vi "RESP3 Format Message.vi"(8 "error in (no error)":errorcluster, 11 "RESP3 Value":variant) -> (0 "error out":errorcluster, 3 "messages":string[](array[string]))   [LabVIEW 2019, in "RESP3.lvlib"]
doc: "<b>Description</b> This VI formats a RESP3 Value into an array of strings that represent the input value. The output of this VI is suitable to send to a peer over a TCP connection.\n\n<b>Inputs</b>\n<b>RESP3 Value</b>: Any valid RESP3 value.\n\n<b>Outputs</b>\n<b>messages</b>: An array of \\r\\n terminated messages that represent the input value.\n\nBSD 3-Clause License\n\nCopyright (c) 2021, TauTerra, LLC\nAll rights reserved.\n\nRedistribution and use in source and binary forms, with or without\nmodification, are permitted provided that the following conditions are met:\n\n1. Redistributions of source code must retain the above copyright notice, this\n list of conditions and the following disclaimer.\n\n2. Redistributions in binary form must reproduce the above copyright notice,\n this list of conditions and the following disclaimer in the documentation\n and/or other materials provided with the distribution.\n\n3. Neither the name of the copyright holder nor the names of its\n contributors may be used to endorse or promote products derived from\n this software without specific prior written permission.\n\nTHIS SOFTWARE IS PROVIDED BY THE COPYRIGHT HOLDERS AND CONTRIBUTORS \"AS IS\"\nAND ANY EXPRESS OR IMPLIED WARRANTIES, INCLUDING, BUT NOT LIMITED TO, THE\nIMPLIED WARRANTIES OF MERCHANTABILITY AND FITNESS FOR A PARTICULAR PURPOSE ARE\nDISCLAIMED. IN NO EVENT SHALL THE COPYRIGHT HOLDER OR CONTRIBUTORS BE LIABLE\nFOR ANY DIRECT, INDIRECT, INCIDENTAL, SPECIAL, EXEMPLARY, OR CONSEQUENTIAL\nDAMAGES (INCLUDING, BUT NOT LIMITED TO, PROCUREMENT OF SUBSTITUTE GOODS OR\nSERVICES; LOSS OF USE, DATA, OR PROFITS; OR BUSINESS INTERRUPTION) HOWEVER\nCAUSED AND ON ANY THEORY OF LIABILITY, WHETHER IN CONTRACT, STRICT LIABILITY,\nOR TORT (INCLUDING NEGLIGENCE OR OTHERWISE) ARISING IN ANY WAY OUT OF THE USE\nOF THIS SOFTWARE, EVEN IF ADVISED OF THE POSSIBILITY OF SUCH DAMAGE."
uses:
  RESP3.lvlib
  types/RESP3 data type attribute.vi
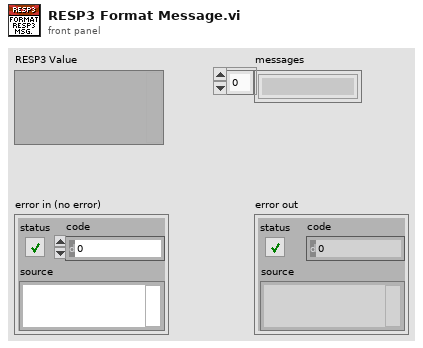
[diagram p1: front panel]
types:
  T1 = typedef "RESP3.lvlib/RESP3 Type.ctl" = enum8{"<0x00>", "<0x01>", "<0x02>", "<0x03>", "<0x04>", "<0x05>", "<0x06>", "<0x07>", "<0x08>", "<0x09>", "<0x0A>", "<0x0B>", "<0x0C>", "<0x0D>", "<0x0E>", "<0x0F>", "<0x10>", "<0x11>", "<0x12>", "<0x13>", "<0x14>", "<0x15>", "<0x16>", "<0x17>", "<0x18>", "<0x19>", "<0x1A>", "<0x1B>", "<0x1C>", "<0x1D>", "<0x1E>", "<0x1F>", "\" \"", "BLOB ERROR", "\"\"\"", "BOOLEAN", "BLOB", "MAP", "\"&\"", "\"'\"", "BIG NUMBER", "\")\"", "ARRAY", "STRING", "DOUBLE", "ERROR", "END", "\"/\"", "\"0\"", "\"1\"", "\"2\"", "\"3\"", "\"4\"", "\"5\"", "\"6\"", "\"7\"", "\"8\"", "\"9\"", "INTEGER", "STREAM", "\"<\"", "VERBATIM STRING", "PUSH", "\"?\"", "\"@\"", "\"A\"", "\"B\"", "\"C\"", "\"D\"", "\"E\"", "\"F\"", "\"G\"", "\"H\"", "\"I\"", "\"J\"", "\"K\"", "\"L\"", "\"M\"", "\"N\"", "\"O\"", "\"P\"", "\"Q\"", "\"R\"", "\"S\"", "\"T\"", "\"U\"", "\"V\"", "\"W\"", "\"X\"", "\"Y\"", "\"Z\"", "\"[\"", "\"\\\"", "\"]\"", "\"^\"", "NULL", "\"`\"", "\"a\"", "\"b\"", "\"c\"", "\"d\"", "\"e\"", "\"f\"", "\"g\"", "\"h\"", "\"i\"", "\"j\"", "\"k\"", "\"l\"", "\"m\"", "\"n\"", "\"o\"", "\"p\"", "\"q\"", "\"r\"", "\"s\"", "\"t\"", "\"u\"", "\"v\"", "\"w\"", "\"x\"", "\"y\"", "\"z\"", "\"{\"", "ATTRIBUTES", "\"}\"", "SET", "<0x7F>", "<0x80>", "<0x81>", "<0x82>", "<0x83>", "<0x84>", "<0x85>", "<0x86>", "<0x87>", "<0x88>", "<0x89>", "<0x8A>", "<0x8B>", "<0x8C>", "<0x8D>", "<0x8E>", "<0x8F>", "<0x90>", "<0x91>", "<0x92>", "<0x93>", "<0x94>", "<0x95>", "<0x96>", "<0x97>", "<0x98>", "<0x99>", "<0x9A>", "<0x9B>", "<0x9C>", "<0x9D>", "<0x9E>", "<0x9F>", "<0xA0>", "<0xA1>", "<0xA2>", "<0xA3>", "<0xA4>", "<0xA5>", "<0xA6>", "<0xA7>", "<0xA8>", "<0xA9>", "<0xAA>", "<0xAB>", "<0xAC>", "<0xAD>", "<0xAE>", "<0xAF>", "<0xB0>", "<0xB1>", "<0xB2>", "<0xB3>", "<0xB4>", "<0xB5>", "<0xB6>", "<0xB7>", "<0xB8>", "<0xB9>", "<0xBA>", "<0xBB>", "<0xBC>", "<0xBD>", "<0xBE>", "<0xBF>", "<0xC0>", "<0xC1>", "<0xC2>", "<0xC3>", "<0xC4>", "<0xC5>", "<0xC6>", "<0xC7>", "<0xC8>", "<0xC9>", "<0xCA>", "<0xCB>", "<0xCC>", "<0xCD>", "<0xCE>", "<0xCF>", "<0xD0>", "<0xD1>", "<0xD2>", "<0xD3>", "<0xD4>", "<0xD5>", "<0xD6>", "<0xD7>", "<0xD8>", "<0xD9>", "<0xDA>", "<0xDB>", "<0xDC>", "<0xDD>", "<0xDE>", "<0xDF>", "<0xE0>", "<0xE1>", "<0xE2>", "<0xE3>", "<0xE4>", "<0xE5>", "<0xE6>", "<0xE7>", "<0xE8>", "<0xE9>", "<0xEA>", "<0xEB>", "<0xEC>", "<0xED>", "<0xEE>", "<0xEF>", "<0xF0>", "<0xF1>", "<0xF2>", "<0xF3>", "<0xF4>", "<0xF5>", "<0xF6>", "<0xF7>", "<0xF8>", "<0xF9>", "<0xFA>", "<0xFB>", "<0xFC>", "<0xFD>", "<0xFE>"}
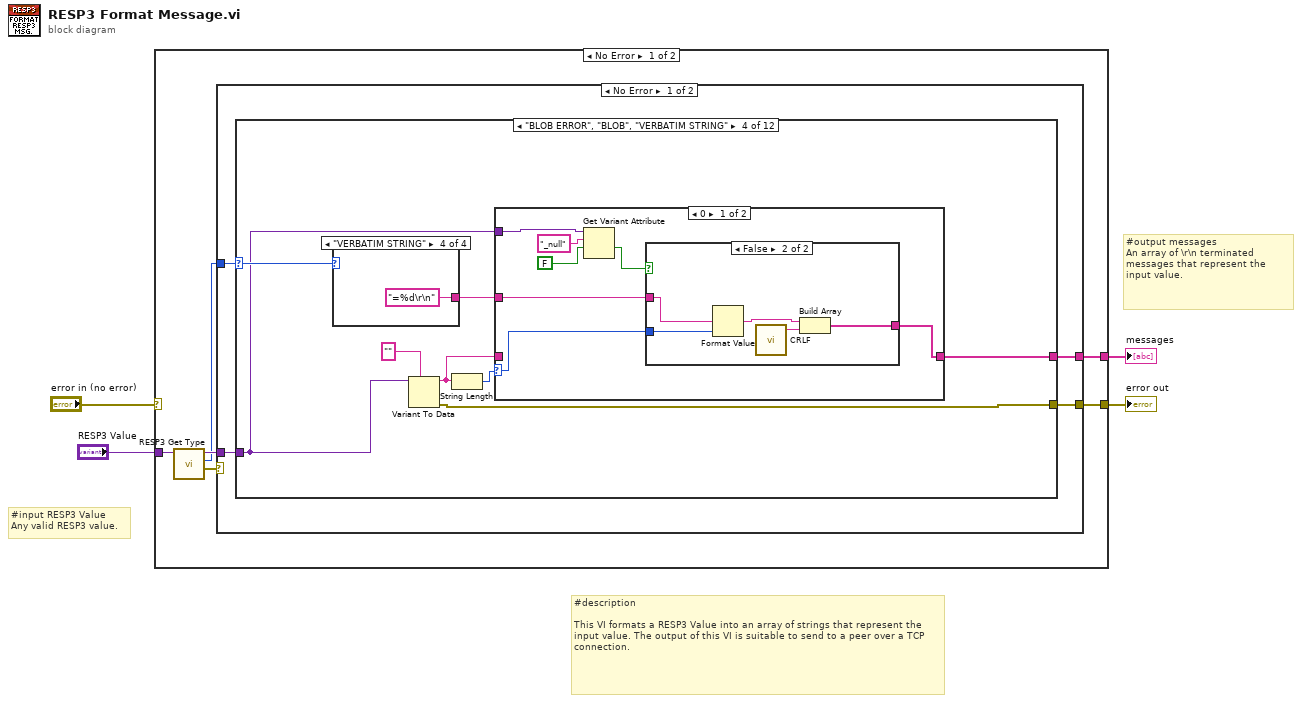
[diagram p0: block diagram]
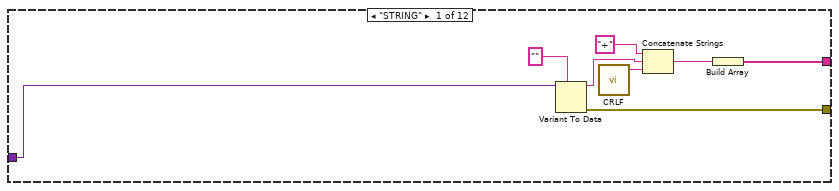
[diagram p2: hidden frame]
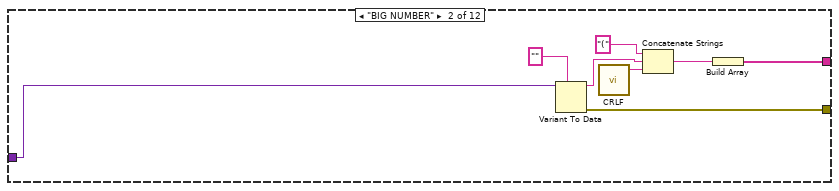
[diagram p3: hidden frame]
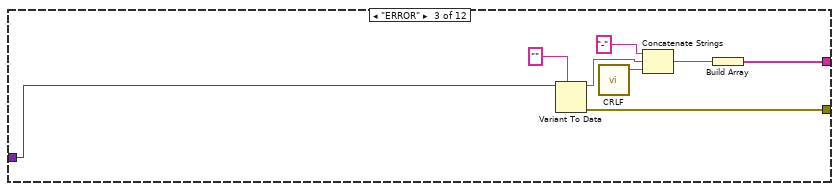
[diagram p4: hidden frame]
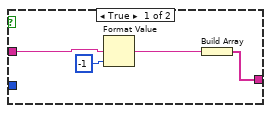
[diagram p5: hidden frame]
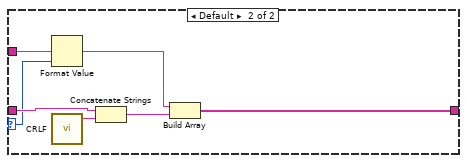
[diagram p6: hidden frame]
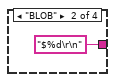
[diagram p8: hidden frame]
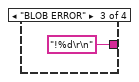
[diagram p9: hidden frame]
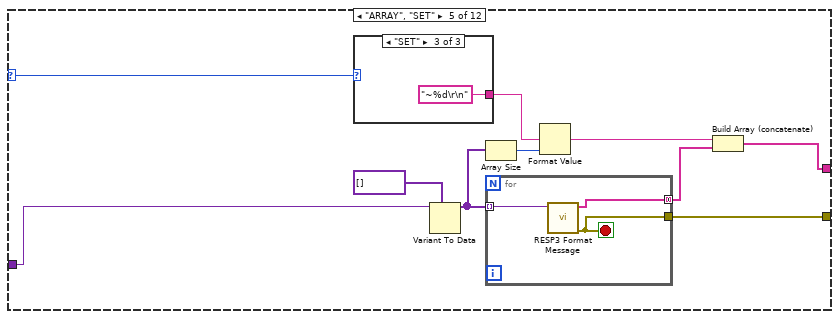
[diagram p10: hidden frame]
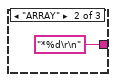
[diagram p12: hidden frame]
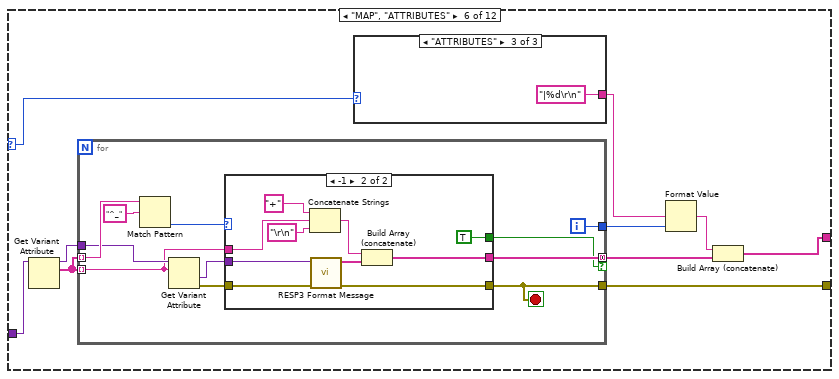
[diagram p13: hidden frame]
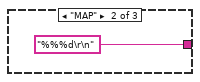
[diagram p15: hidden frame]
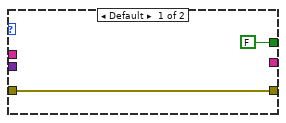
[diagram p16: hidden frame]
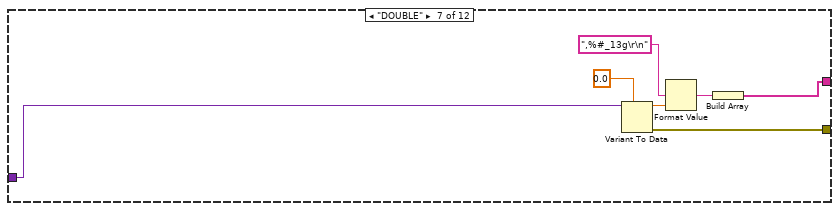
[diagram p17: hidden frame]
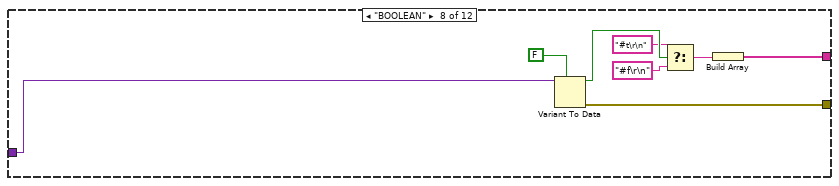
[diagram p18: hidden frame]
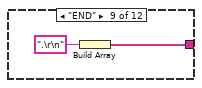
[diagram p19: hidden frame]
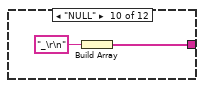
[diagram p20: hidden frame]
diagram:
  # "#description\n\nThis VI formats a RESP3 Value into an array of strings that represent the input value. The output of this VI is suitable to send to a peer over a TCP connection."
  # "#output messages\nAn array of \\r\\n terminated messages that represent the input value."
  # "#input RESP3 Value\nAny valid RESP3 value."
  n1 = case shown="No Error" "error in (no error)" {
    selector: "error in (no error)" -> [_ w152]
    tunnel: "RESP3 Value" -> [w10 _]
    tunnel: [w8 w152] -> w2
    tunnel: [w5 _] -> w1
    frame No Error {
      n2 = call "RESP3 Get Type.vi"("RESP3 Value in"=w10) -> ("error out"=w9:errorcluster, "RESP3 Type"=w6:T1, "RESP3 Value out"=w7:variant)  [unwired: 7 in, 1 out]
      n3 = case shown="No Error" w9 {
        selector: w9 -> [_ w151]
        tunnel: [w12 w151] -> w8
        tunnel: w7 -> [w13 _]
        tunnel: w6 -> [w14 _]
        tunnel: [w11 _] -> w5
        frame No Error {
          n4 = case shown="\"BLOB ERROR\", \"BLOB\", \"VERBATIM STRING\"" w14 {
            selector: w14 -> [_ _ _ w44 w73 w88 _ _ _ _ _ _]
            tunnel: w13 -> [w22 w30 w38 w39 w81 w92 w129 w137 _ _ w148 _]
            tunnel: [w20 w28 w36 w45 w80 w97 w127 w135 _ _ w146 errorcluster {"status"=TRUE, "code"=6015, "source"="invlaid RESP type"} ("error out")] -> w12
            tunnel: [w15 w23 w31 w43 w78 w95 w126 w130 w138 w140 w143 string[] []] -> w11
            frame "STRING" {
              n5 = Variant To Data(type="", Variant=w22) -> (data=w18:string, error out=w20:errorcluster)  [unwired: 1 in]
              n6 = call "CRLF.vi"() -> ("CRLF"=w19:string)  [unwired: 5 in]
              n7 = Concatenate Strings("+" ("string"), w18, w19) -> (w16:string)
              n8 = Build Array(w16) -> (w15:string[])
            }
            frame "BIG NUMBER" {
              n9 = Variant To Data(type="", Variant=w30) -> (data=w26:string, error out=w28:errorcluster)  [unwired: 1 in]
              n10 = call "CRLF.vi"() -> ("CRLF"=w27:string)  [unwired: 5 in]
              n11 = Concatenate Strings("(" ("string"), w26, w27) -> (w24:string)
              n12 = Build Array(w24) -> (w23:string[])
            }
            frame "ERROR" {
              n13 = Variant To Data(type="", Variant=w38) -> (data=w34:string, error out=w36:errorcluster)  [unwired: 1 in]
              n14 = call "CRLF.vi"() -> ("CRLF"=w35:string)  [unwired: 5 in]
              n15 = Concatenate Strings("-" ("string"), w34, w35) -> (w32:string)
              n16 = Build Array(w32) -> (w31:string[])
            }
            frame "BLOB ERROR", "BLOB", "VERBATIM STRING" {
              n17 = case shown="\"VERBATIM STRING\"" w44 {
                tunnel: [_ "$%d\r\n" ("format string") "!%d\r\n" ("format string") "=%d\r\n" ("format string")] -> w40
                frame Default {
                }
                frame "BLOB" {
                }
                frame "BLOB ERROR" {
                }
                frame "VERBATIM STRING" {
                }
              }
              n18 = Variant To Data(type="", Variant=w39) -> (data=w42:string, error out=w45:errorcluster)  [unwired: 1 in]
              n19 = String Length(string=w42) -> (length=w41:i32)
              n20 = case shown="0" w41 {
                selector: w41 -> [w47 w63]
                tunnel: [w52 w67] -> w43
                tunnel: w42 -> [_ w66]
                tunnel: w40 -> [w53 w65]
                tunnel: w39 -> [w51 _]
                frame 0 {
                  n21 = Get Variant Attribute(Variant=w51, name="_null", default value (empty Variant)=FALSE) -> (value=w48:bool)  [unwired: 1 in, 3 out]
                  n22 = case shown="False" w48 {
                    tunnel: w53 -> [w57 w62]
                    tunnel: [w56 w61] -> w52
                    tunnel: w47 -> [_ w59]
                    frame True {
                      n23 = Format Value(format string=w57, value (0)=-1) -> (output string=w55:string)  [unwired: 1 in]
                      n24 = Build Array(w55) -> (w56:string[])
                    }
                    frame False {
                      n25 = Format Value(format string=w62, value (0)=w59) -> (output string=w60:string)  [unwired: 1 in]
                      n26 = call "CRLF.vi"() -> ("CRLF"=w58:string)  [unwired: 5 in]
                      n27 = Build Array(w60, w58) -> (w61:string[])
                    }
                  }
                }
                frame Default {
                  n28 = Format Value(format string=w65, value (0)=w63) -> (output string=w64:string)  [unwired: 1 in]
                  n29 = call "CRLF.vi"() -> ("CRLF"=w69:string)  [unwired: 5 in]
                  n30 = Concatenate Strings(w66, w69) -> (w68:string)
                  n31 = Build Array(w64, w68) -> (w67:string[])
                }
              }
            }
            frame "ARRAY", "SET" {
              n32 = case shown="\"SET\"" w73 {
                tunnel: [_ "*%d\r\n" ("format string") "~%d\r\n" ("format string")] -> w77
                frame Default {
                }
                frame "ARRAY" {
                }
                frame "SET" {
                }
              }
              n33 = Variant To Data(type=variant[] [], Variant=w81) -> (data=w76:variant[])  [unwired: 1 in, 1 out]
              n34 = Array Size(array=w76) -> (size(s)=w75:i32)
              n35 = for {
                tunnel: w76 -> [w87] mode=indexing
                tunnel: [w86] -> w79 mode=concatenating
                tunnel: [w85] -> w80
                stop <- w85 stop-if-true
                n36 = call "RESP3 Format Message.vi"("RESP3 Value"=w87) -> ("error out"=w85:errorcluster, "messages"=w86:string[])  [unwired: 9 in]
              }
              n37 = Format Value(format string=w77, value (0)=w75) -> (output string=w74:string)  [unwired: 1 in]
              n38 = Build Array (concatenate)(w74, w79) -> (w78:string[])
            }
            frame "MAP", "ATTRIBUTES" {
              n39 = Get Variant Attribute(Variant=w92) -> (duplicate Variant=w90:variant, names=w89:string[])  [unwired: 3 in, 2 out]
              n40 = for {
                tunnel: [w110] -> w96 mode=concatenating if=w105
                tunnel: [w109] -> w97
                tunnel: w89 -> [w108] mode=indexing
                tunnel: [w104] -> w91
                tunnel: w90 -> [w103]
                tunnel: w89 -> [w100] mode=indexing
                i -> [w104]
                stop <- w109 stop-if-true
                n41 = Match Pattern(string=w108, regular expression="^_") -> (offset past match=w106:i32)  [unwired: 1 in, 3 out]
                n42 = Get Variant Attribute(Variant=w103, name=w100) -> (value=w102:variant, error out=w101:errorcluster)  [unwired: 2 in, 2 out]
                n43 = case shown="-1" w106 {
                  tunnel: [_ w117] -> w110
                  tunnel: [w111 w121] -> w109
                  tunnel: w102 -> [_ w120]
                  tunnel: [FALSE TRUE] -> w105
                  tunnel: w101 -> [w111 w118]
                  tunnel: w100 -> [_ w114]
                  frame Default {
                  }
                  frame -1 {
                    n44 = Concatenate Strings("+" ("string"), w114, "\r\n" ("string")) -> (w113:string)
                    n45 = call "RESP3 Format Message.vi"("error in (no error)"=w118, "RESP3 Value"=w120) -> ("error out"=w121:errorcluster, "messages"=w122:string[])  [unwired: 8 in]
                    n46 = Build Array (concatenate)(w113, w122) -> (w117:string[])
                  }
                }
              }
              n47 = case shown="\"ATTRIBUTES\"" w88 {
                tunnel: [_ "%%%d\r\n" ("format string") "|%d\r\n" ("format string")] -> w94
                frame Default {
                }
                frame "MAP" {
                }
                frame "ATTRIBUTES" {
                }
              }
              n48 = Format Value(format string=w94, value (0)=w91) -> (output string=w93:string)  [unwired: 1 in]
              n49 = Build Array (concatenate)(w93, w96) -> (w95:string[])
            }
            frame "DOUBLE" {
              n50 = Variant To Data(type=0.0, Variant=w129) -> (data=w124:dbl, error out=w127:errorcluster)  [unwired: 1 in]
              n51 = Format Value(format string=",%#_13g\r\n", value (0)=w124) -> (output string=w123:string)  [unwired: 1 in]
              n52 = Build Array(w123) -> (w126:string[])
            }
            frame "BOOLEAN" {
              n53 = Variant To Data(type=FALSE, Variant=w137) -> (data=w134:bool, error out=w135:errorcluster)  [unwired: 1 in]
              n54 = Select(t="#t\r\n" ("string"), s=w134, f="#f\r\n" ("string")) -> (s? t:f=w131:string)
              n55 = Build Array(w131) -> (w130:string[])
            }
            frame "END" {
              n56 = Build Array(".\r\n" ("string")) -> (w138:string[])
            }
            frame "NULL" {
              n57 = Build Array("_\r\n" ("string")) -> (w140:string[])
            }
            frame "INTEGER" {
              n58 = Variant To Data(type=i64 0, Variant=w148) -> (data=w142:i64, error out=w146:errorcluster)  [unwired: 1 in]
              n59 = Format Value(format string=":%d\r\n", value (0)=w142) -> (output string=w144:string)  [unwired: 1 in]
              n60 = Build Array(w144) -> (w143:string[])
            }
            frame Default {
            }
          }
        }
        frame Error {
        }
      }
    }
    frame Error {
    }
  }
  "error out" <- w2
  "messages" <- w1
